vi "N-Parametric Double FFT Mesurament Test.vi"() -> ()   [LabVIEW 2014]
uses:
  <vilib>/Platform/TimedLoop/XDataNode/timing_clust.ctl
  <vilib>/Platform/TimedLoop/XDataNode/nitl_modes.ctl
  <vilib>/Platform/TimedLoop/XDataNode/wakeup.ctl
  <vilib>/rvi/Analysis/measure/FFT/simModelSupport/niFPGA FFT Streaming Sim Properties.ctl
  <vilib>/rvi/Analysis/measure/FFT/simModelSupport/niFPGA FFT Sim Stream Group Properties.ctl
  <vilib>/rvi/Analysis/measure/FFT/simModelSupport/niFPGA FFT Sim Types.ctl
  <vilib>/rvi/Analysis/measure/FFT/simModelSupport/niFpgaFFTSimArithmeticProperties.ctl
  <vilib>/rvi/Analysis/measure/FFT/simModelSupport/niFpgaFFTSimDfxp.ctl
  <vilib>/fxp/LVFixedPointQuantizationPolicyTypeDef.ctl
  <vilib>/rvi/Analysis/measure/FFT/XNode/niFpgaFFTButterflyDelays.ctl
  <vilib>/rvi/Emulation/niFpgaSctlEmulationGetInTimedLoop.vi
  <vilib>/rvi/Emulation/niFpgaEmulationReportErrorSimple.vi
  <vilib>/rvi/Emulation/niFpgaGetClockAttributes.vi
  <vilib>/rvi/Emulation/niFpgaCriticalErrorInLSC.vi
  <vilib>/rvi/Emulation/niFpgaEmulationIsFPGAContextNoSignature.vi
  <vilib>/rvi/DataTransferAndStorage/Container/Common/niFpgaContainerGetUniqueNameForEmu.vi
  <vilib>/rvi/Memory/Memory_Emulation/niFpgaMemoryEmulationCacheClearOnFirstRun.vi
  <vilib>/rvi/Memory/Memory_Emulation/nirvimemoryEmulationManagerCache_MakeExclusive.vi
  <vilib>/rvi/Memory/Memory_Emulation/niFpgaMemoryEmulationValidateCache.vi
  <vilib>/rvi/Memory/Memory_Emulation/nirvimemoryEmulationManagerCache_InsertValue.vi
  <vilib>/Utility/error.llb/Clear Errors.vi
  <vilib>/rvi/Memory/Memory_Emulation/nirvimemoryEmulationManagerCache_ReleaseExclusive.vi
  <vilib>/rvi/Memory/Memory_Emulation/nirvimemoryEmulationManagerCache_GetValue.vi
  <vilib>/rvi/Memory/Memory_Emulation/nirvimemoryEmulationManagerCache_SetValue.vi
  <vilib>/rvi/Emulation/niFpgaProcessEmulError.vi
  <vilib>/rvi/errors/niFpgaSetErrorForExecOnDevCompSimple.vi
  <vilib>/rvi/eio/common/nirviEmuReportErrorAndStop.vi
  <vilib>/rvi/FIFO/Fifo_Resource/nirvififoEmulationSetSize.vi
  <vilib>/rvi/FIFO/Fifo_Resource/nirviFifoEmulationQueueMgr.vi
  <instcachedir>/0/nirviFifoEmulationQueueMgr_E5CAEC123FF24DC58D834DCA3CDAA9B5.lvgen/nirviFifoEmulationQueueMgr_E5CAEC123FF24DC58D834DCA3CDAA9B5_010.vi
  <vilib>/rvi/FIFO/Fifo_Resource/nirvififoEmulationCreateLock.vi
  <vilib>/rvi/FIFO/Fifo_Resource/nirvififoEmulationObtainLock.vi
  <vilib>/rvi/FIFO/Fifo_Resource/nirvififoEmulationReleaseLock.vi
  <vilib>/rvi/occurrence/nirviWaitOnOccurrenceBase.vi
  <vilib>/rvi/errors/nirviReportUnexpectedCaseInternalError.vi
  <vilib>/rvi/errors/nirviReportUnexpectedCaseInternalError (U32).vi
  <vilib>/rvi/FIFO/Fifo_Resource/nirvififoEmulationDetermineInputValidOut.vi
  <vilib>/rvi/Memory/Memory_Emulation/nirvimemoryFastEmulation.vi
  <vilib>/rvi/Memory/Memory_Emulation/nirvimemoryEmulation.vi
  <vilib>/rvi/eio/common/nirviEmuTemplateMethod_errors.vi
  <vilib>/rvi/Analysis/measure/FFT/simModelSupport/niFpgaFFTSimModelStreamingCore.vi
  <vilib>/rvi/interface/RandomDataEmulation/niFpgaRandomDataHandleErrors.vi
  <vilib>/Platform/TimedLoop/XDataNode/XDataNode.xnode
  <vilib>/rvi/DataTransferAndStorage/Container/XNode/niFpgaContainer.xnode
  <vilib>/rvi/DataTransferAndStorage/Register/Emulation/niFpgaRegisterEmulation.vi
  <vilib>/rvi/FIFO/Fifo_Resource/nirvififoEmulationRead.vi
  <vilib>/rvi/FIFO/Fifo_Resource/nirvififoEmulationWrite.vi
  <vilib>/eio/EIOMethodNode/EIOMethodNode.xnode
  <vilib>/rvi/Analysis/measure/FFT/XNode/niFpgaFFT.xnode
  <vilib>/rvi/interface/RandomDataEmulation/nirviRandomDataFpgaReadWriteTemplate.vi
  <vilib>/Platform/TimedLoop/XDataNode/XDNodeRunTimeDep.lvlib
panel:
  in  "n":u32=1
  in  "Latency points":u32
  in  "snapshot":bool
  in  "lower limit 2":u32=682
  in  "lower limit 1":u32=57
  in  "upper limit 2":u32=1193
  in  "upper limit 1":u32=568
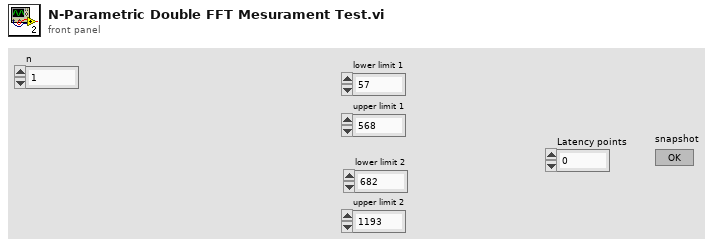
[diagram p1: front panel]
types:
  T1 = typedef "XDNodeRunTimeDep.lvlib/timing_clust.ctl" = cluster{"Expected End [f-1]":u64, "Actual End [f-1]":u64, "Finished Late? [f-1]":bool, "Expected End [i-1]":u64, "Actual End [i-1]":u64, "Finished Late? [i-1]":bool, "Expected Start [i]":u64, "Actual Start [i]":u64, "Expected Start [f]":u64, "Actual Start [f]":u64, "Source Name":string, "Structure Name":string, "Period":i64, "Deadline":i64, "Offset":i64, "Start":i64, "Priority":i32, "Timeout":i32, "Mode":T2, "Wakeup Reason":T3, "Error":errorcluster, "Source Type":string, "Secondary Source Type":string, "Global End Time":u64, "Global Start Time":u64, "Frame Duration":u64, "Iteration Duration":u64, "Assigned CPU":i32, "I/O Scan Engine Mode":u32}
  T2 = typedef "XDNodeRunTimeDep.lvlib/nitl_modes.ctl" = enum32{"No Change", "Process missed periods, maintain original phase", "Discard missed periods, maintain original phase", "Process missed periods, ignore original phase", "Discard missed periods, ignore original phase"}
  T3 = typedef "XDNodeRunTimeDep.lvlib/wakeup.ctl" = enum32{"Normal", "Aborted", "Asynchronous wakeup", "Timing source error", "Timed loop error", "Timeout"}
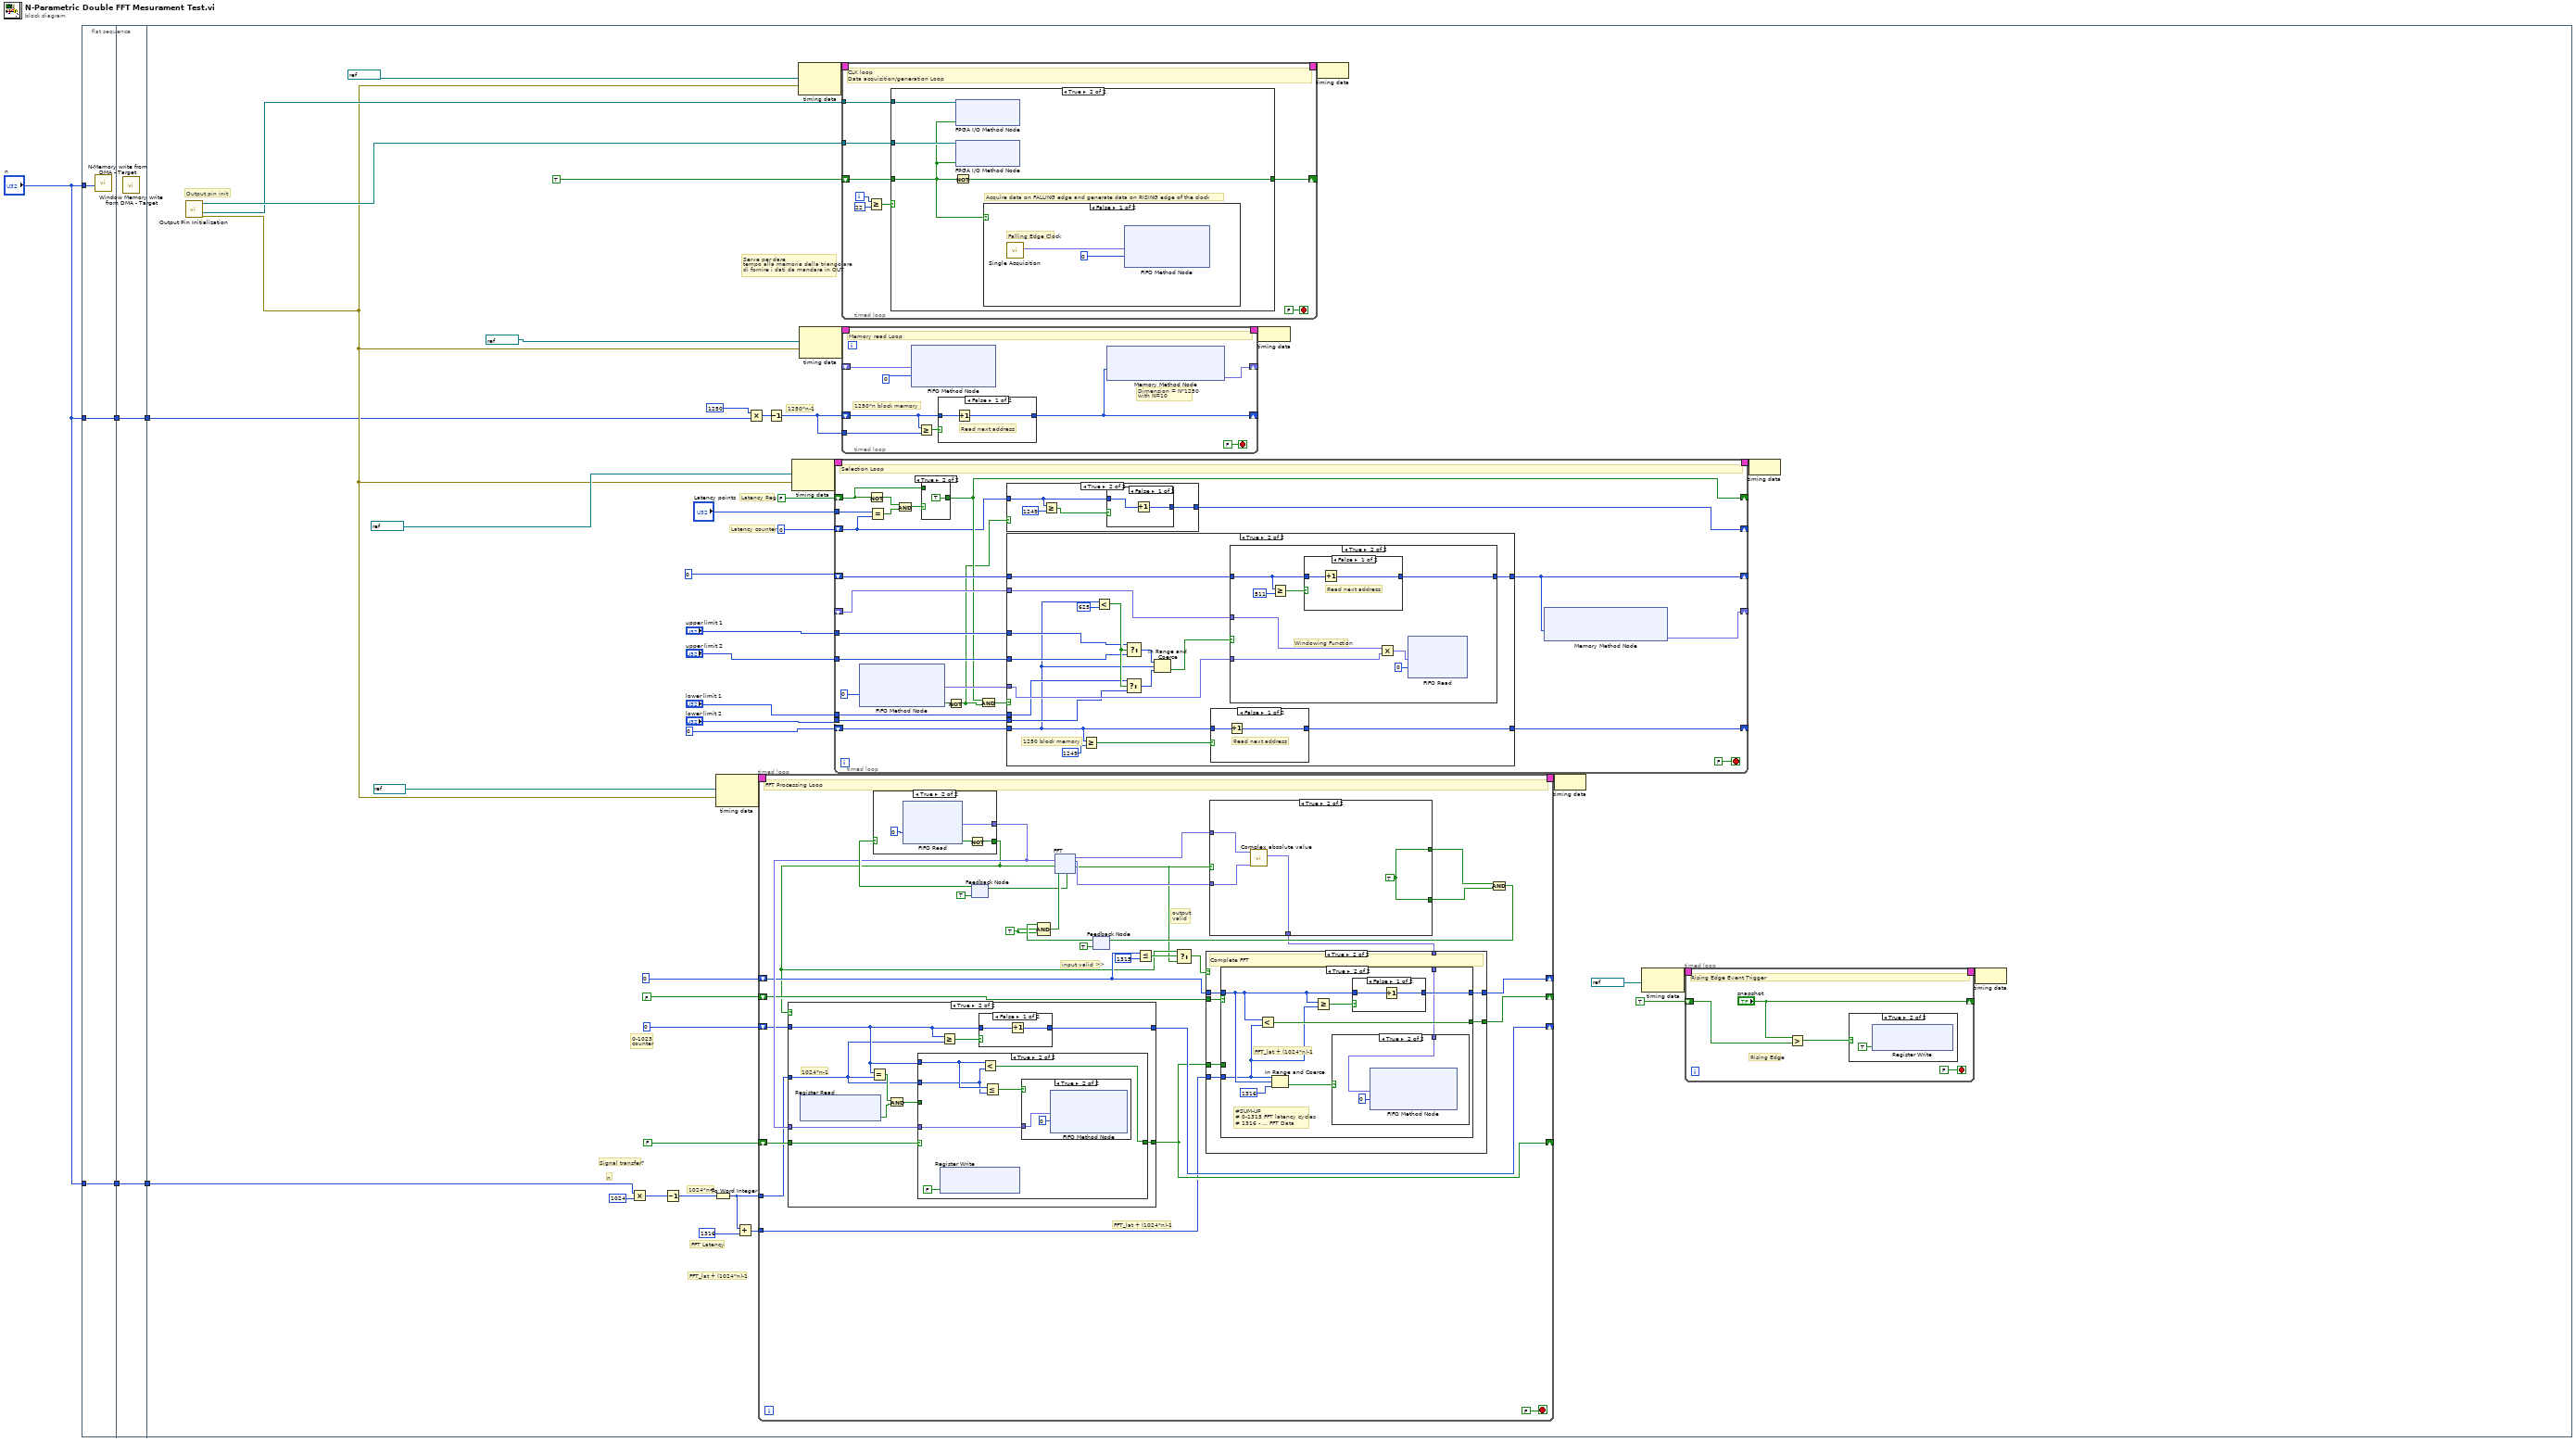
[diagram p0: block diagram]
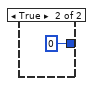
[diagram p4: hidden frame]
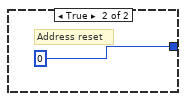
[diagram p8: hidden frame]
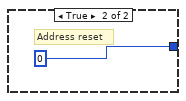
[diagram p9: hidden frame]
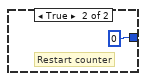
[diagram p13: hidden frame]
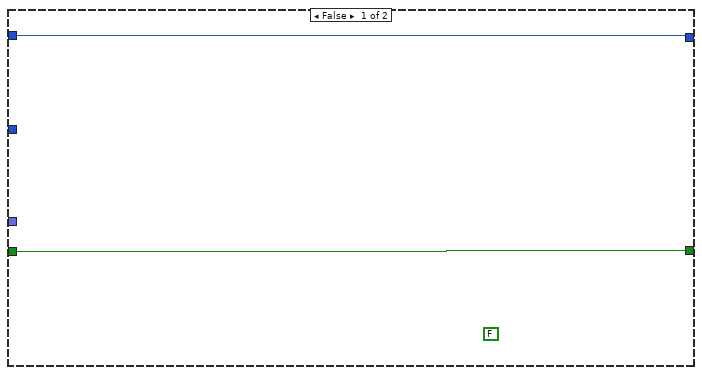
[diagram p14: hidden frame]
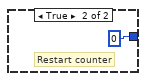
[diagram p17: hidden frame]
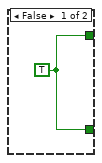
[diagram p18: hidden frame]
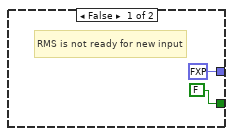
[diagram p19: hidden frame]
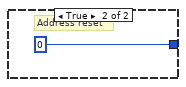
[diagram p20: hidden frame]
diagram:
  n1 = flat-sequence {
    tunnel: "n" -> [w8]
    tunnel: [w7] -> w5
    tunnel: "n" -> [w7]
    tunnel: "n" -> [w6]
    tunnel: [w6] -> w2
    tunnel: w5 -> [w10]
    tunnel: [w10] -> w4
    tunnel: w2 -> [w9]
    tunnel: [w9] -> w1
    tunnel: w4 -> [w20]
    tunnel: w1 -> [w11]
    frame #0 {
      n2 = call "N-Memory write from DMA - Target.vi"("n"=w8) -> ()  [unwired: 11 in]
    }
    frame #1 {
      n3 = call "Window Memory write from DMA - Target.vi"() -> ()  [unwired: 12 in]
    }
    frame #2 {
      # "1250*n-1"
      # "FFT_lat + (1024*n)-1"
      # "FFT Latency"
      # "n"
      # "1024*n-1"
      # "Serve per dare\ntempo alla memoria della triangolare\ndi fornire i dati da mandare in OUT"
      # "Latency counter"
      # "Latency Reg"
      # "0-1023\ncounter"
      # "Signal transfer?"
      # "Output pin init"
      n4 = call "Output Pin Initialization.vi"() -> ("error out"=w38:errorcluster, "I/O Out Clock DAC (pin16)"=w42:refnum<k21>, "I/O Out Clock ADC (pin17)"=w43:refnum<k21>)  [unwired: 8 in]
      n5 = Multiply(x=w20, y=u32 1024) -> (x*y=w21:u32)
      n6 = Decrement(x=w21) -> (x-1=w19:u32)
      n7 = To Word Integer(number=w19) -> (16bit integer=w17:i16)
      n8 = node-c288(refnum<k21> "40MHz" ("Source Name"), w38) -> (w50:T1)
      n9 = Add(x=w17, y=i16 1316) -> (x+y=w15:i16)
      n10 = Multiply(x=u32 1250, y=w11) -> (x*y=w13:u32)
      n11 = timed-loop {
        timing: w50 -> [_]
        timing-out: [_] -> w49
        shift-right: [w154] -> _
        shift-left: FALSE -> [w157]
        shift-right: [w158] -> _
        shift-left: i16 0 -> [w155]
        shift-right: [w153] -> _
        shift-left: FALSE -> [w152]
        shift-right: [w151] -> _
        shift-left: i16 0 -> [w149]
        tunnel: w17 -> [w142]
        tunnel: w15 -> [w141]
        stop <- FALSE stop-if-true
        w143 = TRUE
        # "FFT_lat + (1024*n)-1"
        # "output\nvalid"
        # "input valid >>"
        # "FFT Processing Loop"
        n12 = feedback #1(TRUE ("ready for input")) -> (w170:bool)
        n13 = case shown="True" w170 {
          tunnel: [FALSE w255] -> w145
          tunnel: [fxp<+/-,12,12> 0.0 ("Element") w252] -> w156
          frame False {
            # "RMS is not ready for new input"
          }
          frame True {
            n14 = xnode ("FIFO Read")("Timeout"=0) -> ("Element"=w252:fxp<+/-,12,12>, "Timed Out?"=w254:bool)  [unwired: 1 in, 1 out]
            n15 = Not(x=w254) -> (.not. x?=w255:bool)
          }
        }
        n16 = case shown="True" w145 {
          tunnel: w155 -> [w196 w202]
          tunnel: [w196 w205] -> w158
          tunnel: w157 -> [w195 w200]
          tunnel: [w195 w201] -> w154
          tunnel: w156 -> [_ w199]
          tunnel: w142 -> [_ w197]
          frame False {
            (unwired) FALSE
          }
          frame True {
            # "1024*n-1"
            n17 = xnode ("Register Read")() -> ("Data"=w198:bool)  [unwired: 1 in, 1 out]
            n18 = Equal?(x=w202, y=w197) -> (x = y?=w204:bool)
            n19 = And(x=w204, y=w198) -> (x .and. y?=w203:bool)
            n20 = case shown="True" w200 {
              tunnel: w203 -> [w207 _]
              tunnel: w202 -> [_ w209]
              tunnel: [w207 w213] -> w201
              tunnel: w199 -> [_ w211]
              tunnel: w197 -> [_ w208]
              frame False {
              }
              frame True {
                n21 = xnode ("Register Write")("Data"=FALSE) -> ()  [unwired: 1 in, 1 out]
                n22 = Less?(x=w209, y=w208) -> (x < y?=w213:bool)
                n23 = Less Or Equal?(x=w209, y=w208) -> (x <= y?=w212:bool)
                n24 = case shown="True" w212 {
                  tunnel: w211 -> [_ w214]
                  frame False {
                  }
                  frame True {
                    n25 = xnode ("FIFO Method Node")("Element"=w214, "Timeout"=0) -> ()  [unwired: 1 in, 2 out]
                  }
                }
              }
            }
            n26 = Greater Or Equal?(x=w202, y=w197) -> (x >= y?=w206:bool)
            n27 = case shown="False" w206 {
              tunnel: w202 -> [w217 _]
              tunnel: [w216 i16 0] -> w205
              frame False {
                n28 = Increment(x=w217) -> (x+1=w216:i16)
              }
              frame True {
                # "Restart counter"
              }
            }
          }
        }
        n29 = feedback #2(TRUE) -> (w166:bool)
        n30 = Compound Arithmetic op=AND(w166, w143, w143) -> (w165:bool)
        n31 = xnode "FFT"("real data in"=w156, "input valid"=w145, "ready for output"=w165) -> ("ready for input"=w164:bool, "real data out"=w163:fxp<+/-,22,22>, "imaginary data out"=w162:fxp<+/-,22,22>, "output valid"=w144:bool)  [unwired: 2 in, 1 out]
        n32 = feedback-in #1(w164) -> ()
        n33 = Less Or Equal?(x=w149, y=i16 1315) -> (x <= y?=w150:bool)
        n34 = Select(t=w145, s=w150, f=w144) -> (s? t:f=w147:bool)
        n35 = case shown="True" w144 {
          tunnel: w163 -> [_ w249]
          tunnel: w162 -> [_ w248]
          tunnel: [w245 w246] -> w161
          tunnel: [w245 w246] -> w160
          tunnel: [_ w247] -> w146
          frame False {
            w245 = TRUE
          }
          frame True {
            w246 = TRUE
            n36 = call "Complex absolute value.vi"("Im"=w248, "Re"=w249) -> ("Square Absolute Value"=w247:fxp<+,44,44>)  [unwired: 9 in]
          }
        }
        n37 = case shown="True" w147 {
          tunnel: w154 -> [_ w179]
          tunnel: [w171 w178] -> w153
          tunnel: w152 -> [w171 w177]
          tunnel: w149 -> [w172 w176]
          tunnel: [w172 w175] -> w151
          tunnel: w146 -> [_ w174]
          tunnel: w141 -> [_ w173]
          frame False {
          }
          frame True {
            # "Complete FFT"
            n38 = case shown="True" w177 {
              tunnel: w179 -> [w181 _]
              tunnel: [w181 w189] -> w178
              tunnel: w176 -> [w180 w185]
              tunnel: [w180 w187] -> w175
              tunnel: w174 -> [_ w183]
              tunnel: w173 -> [_ w182]
              frame False {
              }
              frame True {
                # "FFT_lat + (1024*n)-1"
                # "#SUM-UP\n# 0-1315 FFT latency cycles\n# 1316 - ... FFT Data"
                n39 = Less?(x=w185, y=w182) -> (x < y?=w189:bool)
                n40 = In Range and Coerce(upper limit=w182, x=w185, lower limit=i16 1316 ("y")) -> (In Range?=w184:bool)  [unwired: 1 out]
                n41 = Greater Or Equal?(x=w185, y=w182) -> (x >= y?=w188:bool)
                n42 = case shown="True" w184 {
                  tunnel: w183 -> [_ w191]
                  frame False {
                  }
                  frame True {
                    n43 = xnode ("FIFO Method Node")("Element"=w191, "Timeout"=0) -> ()  [unwired: 1 in, 2 out]
                  }
                }
                n44 = case shown="False" w188 {
                  tunnel: w185 -> [w193 _]
                  tunnel: [w192 i16 0] -> w187
                  frame False {
                    n45 = Increment(x=w193) -> (x+1=w192:i16)
                  }
                  frame True {
                    # "Restart counter"
                  }
                }
              }
            }
          }
        }
        n46 = Compound Arithmetic op=AND(w161, w160) -> (w159:bool)
        n47 = feedback-in #2(w159) -> ()
      }
      n48 = Decrement(x=w13) -> (x-1=w12:u32)
      n49 = node-c288(refnum<k21> "40MHz" ("Source Name"), w38) -> (w48:T1)
      n50 = node-c288(refnum<k21> "80MHz" ("Source Name"), w38) -> (w54:T1)
      n51 = node-c288(refnum<k21> "40MHz" ("Source Name"), w38) -> (w52:T1)
      n52 = timed-loop {
        timing: w48 -> [_]
        timing-out: [_] -> w47
        shift-right: [w88] -> _
        shift-left: u32 0 -> [w75]
        tunnel: "upper limit 1" -> [w84]
        tunnel: "upper limit 2" -> [w83]
        tunnel: "lower limit 1" -> [w82]
        tunnel: "lower limit 2" -> [w81]
        shift-right: [w77] -> _
        shift-left: u32 0 -> [w80]
        shift-right: [w78] -> _
        shift-left: _ -> [w79]
        shift-right: [w69] -> _
        shift-left: FALSE -> [w70]
        tunnel: "Latency points" -> [w74]
        shift-right: [w67] -> _
        shift-left: u32 0 -> [w66]
        stop <- FALSE stop-if-true
        # "Selection Loop"
        n53 = xnode ("FIFO Method Node")("Timeout"=0) -> ("Element"=w86:fxp<+/-,12,12>, "Timed Out?"=w87:bool)  [unwired: 1 in, 1 out]
        n54 = Not(x=w70) -> (.not. x?=w73:bool)
        n55 = Equal?(x=w74, y=w66) -> (x = y?=w72:bool)
        n56 = And(x=w73, y=w72) -> (x .and. y?=w71:bool)
        n57 = case shown="True" w71 {
          tunnel: [w98 TRUE] -> w69
          tunnel: w70 -> [w98 _]
          frame False {
          }
          frame True {
          }
        }
        n58 = Not(x=w87) -> (.not. x?=w68:bool)
        n59 = And(x=w69, y=w68) -> (x .and. y?=w76:bool)
        n60 = case shown="True" w68 {
          tunnel: w66 -> [w90 w93]
          tunnel: [w90 w91] -> w67
          frame False {
          }
          frame True {
            n61 = Greater Or Equal?(x=w93, y=u32 1249) -> (x >= y?=w92:bool)
            n62 = case shown="False" w92 {
              tunnel: w93 -> [w96 _]
              tunnel: [w95 u32 0] -> w91
              frame False {
                n63 = Increment(x=w96) -> (x+1=w95:u32)
              }
              frame True {
              }
            }
          }
        }
        n64 = case shown="True" w76 {
          tunnel: [w101 w116] -> w88
          tunnel: w75 -> [w101 w103]
          tunnel: w86 -> [_ w111]
          tunnel: w84 -> [_ w110]
          tunnel: w83 -> [_ w109]
          tunnel: w82 -> [_ w108]
          tunnel: w81 -> [_ w107]
          tunnel: w80 -> [w100 w104]
          tunnel: [w100 w106] -> w77
          tunnel: w79 -> [_ w105]
          frame False {
          }
          frame True {
            # "1250 block memory"
            n65 = Greater Or Equal?(x=w103, y=u32 1249) -> (x >= y?=w117:bool)
            n66 = Less?(x=w103, y=u32 625) -> (x < y?=w112:bool)
            n67 = Select(t=w108, s=w112, f=w107) -> (s? t:f=w114:u32)
            n68 = Select(t=w110, s=w112, f=w109) -> (s? t:f=w115:u32)
            n69 = In Range and Coerce(upper limit=w115, x=w103, lower limit=w114) -> (In Range?=w102:bool)  [unwired: 1 out]
            n70 = case shown="False" w117 {
              tunnel: w103 -> [w132 _]
              tunnel: [w131 u32 0] -> w116
              frame False {
                # "Read next address"
                n71 = Increment(x=w132) -> (x+1=w131:u32)
              }
              frame True {
                # "Address reset"
              }
            }
            n72 = case shown="True" w102 {
              tunnel: w111 -> [_ w120]
              tunnel: w104 -> [w119 w125]
              tunnel: [w119 w127] -> w106
              tunnel: w105 -> [_ w123]
              frame False {
              }
              frame True {
                # "Windowing Function"
                n73 = Greater Or Equal?(x=w125, y=u32 511) -> (x >= y?=w126:bool)
                n74 = case shown="False" w126 {
                  tunnel: w125 -> [w129 _]
                  tunnel: [w128 u32 0] -> w127
                  frame False {
                    # "Read next address"
                    n75 = Increment(x=w129) -> (x+1=w128:u32)
                  }
                  frame True {
                    # "Address reset"
                  }
                }
                n76 = Multiply(x=w123, y=w120) -> (x*y=w121:fxp<+/-,12,12>)
                n77 = xnode ("FIFO Read")("Element"=w121, "Timeout"=0) -> ()  [unwired: 1 in, 2 out]
              }
            }
          }
        }
        n78 = xnode ("Memory Method Node")("Address"=w77) -> ("Data"=w78:fxp<+,8,1>)  [unwired: 1 in, 1 out]
      }
      n79 = timed-loop {
        timing: w54 -> [_]
        timing-out: [_] -> w53
        shift-right: [w286] -> _
        shift-left: TRUE -> [w284]
        tunnel: w42 -> [w288]
        tunnel: w43 -> [w285]
        i -> [w282]
        stop <- FALSE stop-if-true
        # "CLK loop\nData acquisition/generation Loop"
        n80 = Greater Or Equal?(x=w282, y=22) -> (x >= y?=w281:bool)
        n81 = case shown="True" w281 {
          tunnel: w288 -> [_ w293]
          tunnel: [w289 w292] -> w286
          tunnel: w285 -> [_ w291]
          tunnel: w284 -> [w289 w290]
          frame False {
          }
          frame True {
            # "Acquire data on FALLING edge and generate data on RISING edge of the clock"
            n82 = Not(x=w290) -> (.not. x?=w292:bool)
            n83 = xnode "FPGA I/O Method Node"("FPGA I/O In"=w293, "Data"=w290) -> ()  [unwired: 1 out]
            n84 = xnode "FPGA I/O Method Node"("FPGA I/O In"=w291, "Data"=w290) -> ()  [unwired: 1 out]
            n85 = case shown="False" w290 {
              frame False {
                # "Falling Edge Clock"
                n86 = call "Single Acquisition.vi"() -> ("Out"=w295:fxp<+/-,12,12>)  [unwired: 10 in, 1 out]
                n87 = xnode ("FIFO Method Node")("Element"=w295, "Timeout"=0) -> ()  [unwired: 1 in, 2 out]
              }
              frame True {
                # "Rising Edge Clock"
                n88 = xnode ("FIFO Method Node")("Timeout"=0) -> ("Element"=w296:fxp<+/-,12,12>, "Timed Out?"=w297:bool)  [unwired: 1 in, 1 out]
                n89 = case shown="False" w297 {
                  tunnel: w296 -> [w301 _]
                  frame False {
                    # "Data Generation"
                    n90 = Add(x=w301, y=fxp<+,12,12> 2048.0) -> (x+y=w299:fxp<+/-,14,14>)
                    n91 = call "Single Point Wave generation.vi"("Data To Write"=w299) -> ()  [unwired: 10 in, 1 out]
                  }
                  frame True {
                    # "FPGA memory slow"
                  }
                }
              }
            }
          }
        }
      }
      n92 = timed-loop {
        timing: w52 -> [_]
        timing-out: [_] -> w51
        shift-right: [w264] -> _
        shift-left: w12 -> [w268]
        shift-right: [w266] -> _
        shift-left: _ -> [w265]
        tunnel: w12 -> [w263]
        stop <- FALSE stop-if-true
        # "Dimension = N*1250\nwith N=10"
        # "1250*n block memory"
        # "Memory read Loop"
        n93 = xnode ("FIFO Method Node")("Element"=w265, "Timeout"=0) -> ()  [unwired: 1 in, 2 out]
        n94 = Greater Or Equal?(x=w268, y=w263) -> (x >= y?=w270:bool)
        n95 = case shown="False" w270 {
          tunnel: w268 -> [w272 _]
          tunnel: [w271 u32 0] -> w264
          frame False {
            # "Read next address"
            n96 = Increment(x=w272) -> (x+1=w271:u32)
          }
          frame True {
            # "Address reset"
          }
        }
        n97 = xnode ("Memory Method Node")("Address"=w264) -> ("Data"=w266:fxp<+/-,12,12>)  [unwired: 1 in, 1 out]
      }
      n98 = node-c288(w51) -> ()
      n99 = node-c288(w53) -> ()
      n100 = node-c288(w49) -> ()
      n101 = node-c288(refnum<k21> "40MHz" ("Source Name")) -> (w28:T1)
      n102 = timed-loop {
        timing: w28 -> [_]
        timing-out: [_] -> w27
        shift-right: ["snapshot"] -> _
        shift-left: TRUE ("snapshot") -> [w57]
        stop <- FALSE stop-if-true
        # "Rising Edge"
        # "Rising Edge Event Trigger"
        n103 = Greater?(x="snapshot", y=w57) -> (0:w55:bool)
        n104 = case shown="True" w55 {
          frame False {
          }
          frame True {
            n105 = xnode ("Register Write")("Data"=TRUE) -> ()  [unwired: 1 in, 1 out]
          }
        }
      }
      n106 = node-c288(w47) -> ()
      n107 = node-c288(w27) -> ()
    }
  }
